vi "Test.vi"() -> ()   [LabVIEW 2012]
doc: "This example shows how to read values from a digital channel.\n\nIt will display the digital value as Low (LED off) or High (LED on).\n\nThis example works with the NI 9403 module connected to a Digital Sidecar. The Digital Sidecar should have 12V applied to the WAGO connector. Note that the digital channels are pulled high when floating. This means that if you want to read a limit switch, you would need to connect one end of the switch to SIG and the other end to (-). The the LED would be On when the switch is open and Off when the switch is closed."
uses:
  <vilib>/Rock Robotics/SystemInterfaces/Typedef/FPGA_TypedefDigitalModule.ctl
  <vilib>/Rock Robotics/WPI/Relay/WPI_RelayDirection.ctl
  <vilib>/Rock Robotics/SystemInterfaces/Utilities/FPGA_UtilitiesLED Source.ctl
  <vilib>/Rock Robotics/SystemInterfaces/Utilities/FPGA_UtilitiesLED State.ctl
  <vilib>/Rock Robotics/WPI/MotorControl/WPI_MotorControlOpen Victor.vi
panel:
  out "PWM":bool[](array[boolean])
  in  "PWM Out":dbl(knob) scale=-1.0..1.0
  in  "Foward":bool
  out "Relay":T1
  out "DIO":bool[](array[boolean])
  out "Beacon\nLight":bool
  in  "DIO Module":T2
  in  "stop":bool
  # "I2C"
  # "Set these inputs before running."
  # "Green/Foward is Signal 5 V"
  # "Red / Reverse is Power 5V"
  # "DIO 1"
  # "DIO 2"
  # "Digital Side Car"
  # "DIO 3"
  # "DIO 4"
  # "DIO 5"
  # "DIO 6"
  # "DIO 7"
  # "DIO 8"
  # "DIO 9"
  # "DIO 10"
  # "DIO 11"
  # "DIO  12"
  # "DIO 13"
  # "DIO 14"
  # "DIO 1"
  # "DIO 2"
  # "DIO 3"
  # "DIO 4"
  # "DIO 5"
  # "DIO 6"
  # "DIO 7"
  # "DIO 8"
  # "DIO 9"
  # "DIO 10"
  # "Reverse"
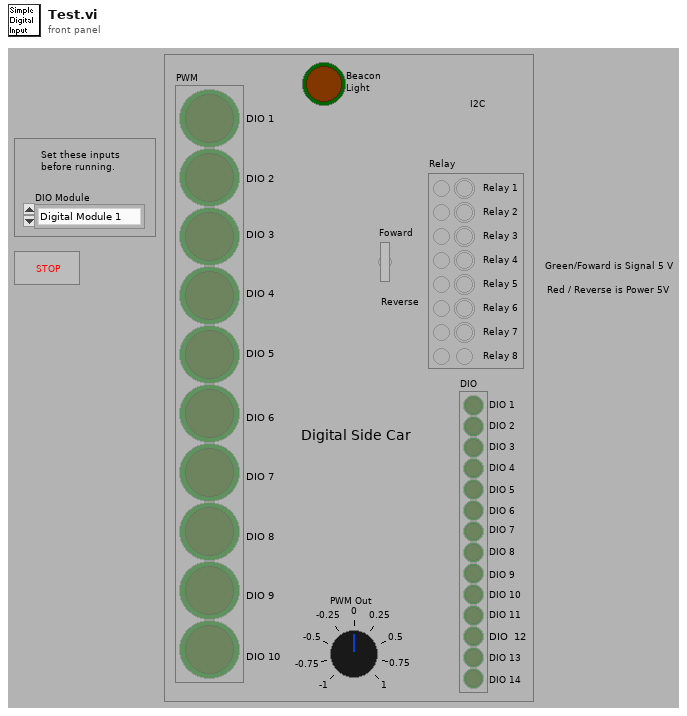
[diagram p1: front panel]
types:
  T1 = cluster{"Relay 1":bool, "Boolean":bool, "Boolean 2":bool, "Relay 2":bool, "Boolean 3":bool, "Relay 3":bool, "Boolean 4":bool, "Relay 4":bool, "Boolean 5":bool, "Relay 5":bool, "Boolean 6":bool, "Relay 6":bool, "Boolean 7":bool, "Relay 7":bool, "Boolean 8":bool, "Relay 8":bool}
  T2 = typedef "FPGA_TypedefDigitalModule.ctl" = enum16{"Digital Module 1", "Digital Module 2"}
  T3 = typedef "WPI_MotorControlDeviceRef.ctl" = cluster{"DeviceStatus":errorcluster, "Type":enum16{"PWM", "CAN"}, "PWM":cluster{"Digital Module":T2, "PWM Channel":T4, "DeadBand":T5}, "CAN":cluster{"Device Number":u8, "Control Mode":T6, "Semaphore":T7, "Max Vout":dbl}, "Invert":bool, "TransformRef":T8, "InvTransformRef":T8}
  T4 = typedef "FPGA_DIOPWMChannel.ctl" = enum8{"PWM 1", "PWM 2", "PWM 3", "PWM 4", "PWM 5", "PWM 6", "PWM 7", "PWM 8", "PWM 9", "PWM 10", "Invalid"}
  T5 = typedef "WPI_PWMDeadband.ctl" = cluster{"Name":string, "maxPositivePwm":i32, "minPositivePwm":i32, "centerPwm":i32, "maxNegativePwm":i32, "minNegativePwm":i32, "angularRange":u16}
  T6 = typedef "WPI_CANJaguar_ControlMode.ctl" = enum8{"Percent VBus", "Current", "Speed", "Position", "Voltage"}
  T7 = typedef "Semaphore RefNum" = refnum<k1>
  T8 = typedef "WPI_PWMTransform_ConPane.ctl" = refnum<vi>
  T9 = typedef "WPI_DigitalInputDevRef.ctl" = cluster{"DevStatus":errorcluster, "DIO Channel":T10, "Digital Module":T2}
  T10 = typedef "FPGA_DIOChannel.ctl" = enum8{"DIO 1", "DIO 2", "DIO 3", "DIO 4", "DIO 5", "DIO 6", "DIO 7", "DIO 8", "DIO 9", "DIO 10", "DIO 11", "DIO 12", "DIO 13", "DIO 14", "Invalid"}
  T11 = typedef "WPI_RelayDirection.ctl" = enum16{"Both directions", "Forward only", "Reverse only"}
  T12 = typedef "WPI_RelayDevRef.ctl" = cluster{"DevStatus":errorcluster, "Relay Channel":T13, "Digital Module":T2, "Relay Direction":T11}
  T13 = typedef "FPGA_DIORelayChannel.ctl" = enum8{"Relay 1", "Relay 2", "Relay 3", "Relay 4", "Relay 5", "Relay 6", "Relay 7", "Relay 8", "Invalid"}
  T14 = typedef "FPGA_UtilitiesLED State.ctl" = enum16{"Off", "On", "Toggle"}
  T15 = typedef "FPGA_UtilitiesLED Source.ctl" = enum16{"User LED", "FPGA LED"}
  T16 = cluster{bool, bool, bool, bool, bool, bool, bool, bool, bool, bool, bool, bool, bool, bool, bool, bool}
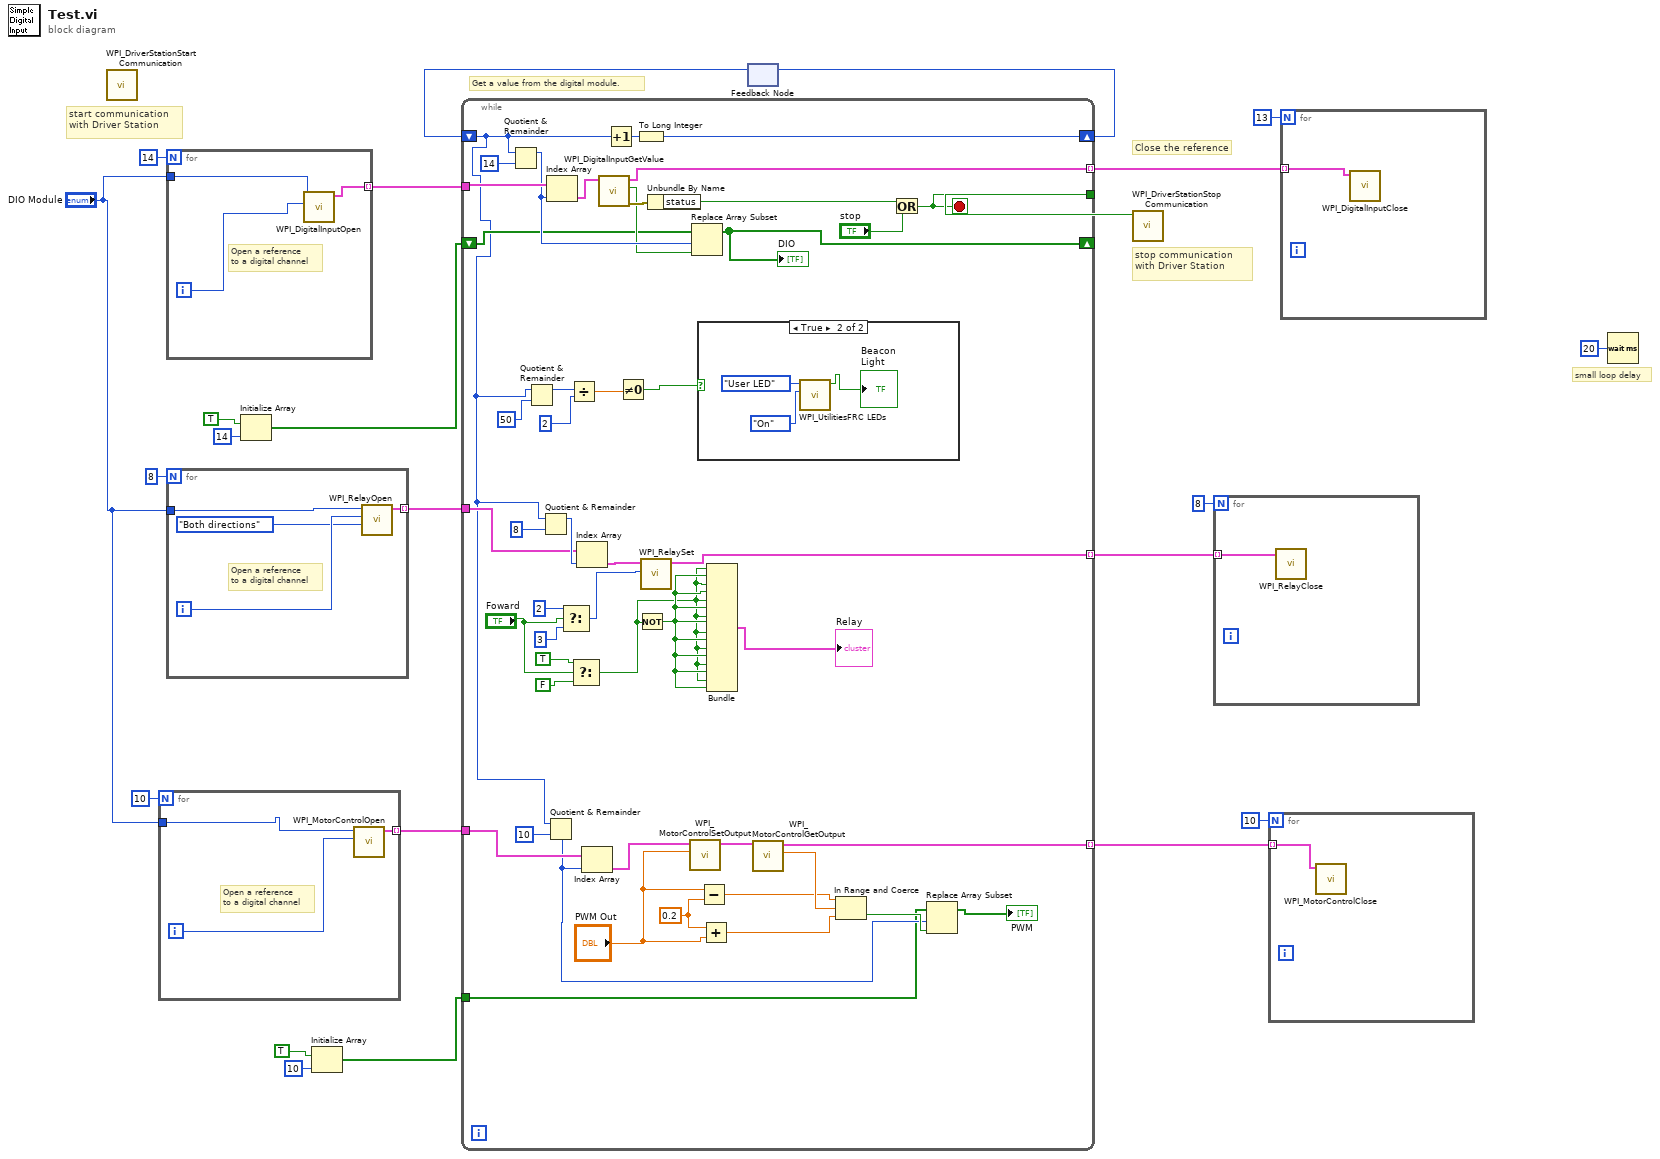
[diagram p0: block diagram]
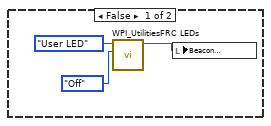
[diagram p2: hidden frame]
diagram:
  # "Get a value from the digital module."
  # "small loop delay"
  # "stop communication with Driver Station"
  # "start communication with Driver Station"
  # "Close the reference"
  n1 = call <vilib>:"WPI_DriverStationStart Communication.vi"() -> ()  [unwired: 1 in, 11 out]
  n2 = for {
    N: 10 -> [_]
    tunnel: [w25] -> w7 mode=indexing
    tunnel: "DIO Module" -> [w24]
    i -> [w26]
    # "Open a reference\nto a digital channel"
    n3 = call-poly <vilib>:"WPI_MotorControlOpen.vi"("PWM Channel"=w26, "Digital Module (Module 1)"=w24) -> ("MotorControlDeviceRef"=w25:T3)  [unwired: 8 in, 1 out]
  }
  n4 = for {
    N: 14 -> [_]
    tunnel: [w29] -> w21 mode=indexing
    tunnel: "DIO Module" -> [w27]
    i -> [w28]
    # "Open a reference\nto a digital channel"
    n5 = call <vilib>:"WPI_DigitalInputOpen.vi"("DIO Channel"=w28, "Digital Module (Module 1)"=w27) -> ("DigitalInputDevRef"=w29:T9)  [unwired: 1 in, 8 out]
  }
  n6 = for {
    N: 8 -> [_]
    tunnel: [w31] -> w11 mode=indexing
    tunnel: "DIO Module" -> [w30]
    i -> [w33]
    # "Open a reference\nto a digital channel"
    n7 = call <vilib>:"WPI_RelayOpen.vi"("Relay Direction"=WPI_RelayDirection."Both directions", "Relay Channel"=w33, "Digital Module (Module 1)"=w30) -> ("RelayDevRef"=w31:T12)  [unwired: 7 in, 1 out]
  }
  n8 = Initialize Array(TRUE, 14 ("dimension size")) -> (w15:bool[])
  n9 = Initialize Array(TRUE, 10 ("dimension size")) -> (w4:bool[])
  n10 = feedback #1() -> (w18:i32)  [unwired: 1 in]
  n11 = while {
    tunnel: [w80] -> w23
    tunnel: w21 -> [w73]
    shift-right: [w75] -> w19
    shift-left: w18 -> [w50]
    shift-right: [w69] -> _
    shift-left: w15 -> [w70]
    tunnel: [w68] -> w13 mode=indexing
    tunnel: w11 -> [w65]
    tunnel: [w57] -> w9 mode=indexing
    tunnel: w7 -> [w49]
    tunnel: w4 -> [w38]
    tunnel: [w34] -> w1 mode=indexing
    stop <- w80 stop-if-true
    w42 = 0.2
    n12 = Quotient & Remainder(x=w50, y=14) -> (x-y*floor(x/y)=w72:i32)  [unwired: 1 out]
    n13 = Quotient & Remainder(x=w50, y=50) -> (x-y*floor(x/y)=w55:i32)  [unwired: 1 out]
    n14 = Quotient & Remainder(x=w50, y=8) -> (x-y*floor(x/y)=w66:i32)  [unwired: 1 out]
    n15 = Quotient & Remainder(x=w50, y=10) -> (x-y*floor(x/y)=w39:i32)  [unwired: 1 out]
    n16 = Index Array(array=w73, index=w72) -> (element=w74:T9)
    n17 = Select(t=2, s="Foward", f=3 ("t")) -> (s? t:f=w61:i32)
    n18 = Divide(x=w55, y=2) -> (x/y=w52:dbl)
    n19 = Select(t=TRUE, s="Foward", f=FALSE) -> (s? t:f=w35:bool)
    n20 = Index Array(array=w65, index=w66) -> (element=w64:T12)
    n21 = Index Array(array=w49, index=w39) -> (element=w48:T3)
    n22 = call <vilib>:"WPI_DigitalInputGetValue.vi"("DigitalInputDevRef"=w74) -> ("error out"=w79:errorcluster, "Value"=w71:bool, "DigitalInputDevRef"=w68:T9)  [unwired: 1 in, 7 out]
    n23 = Increment(x=w50) -> (x+1=w77:i32)
    n24 = Not Equal To 0?(x=w52) -> (x != 0?=w53:bool)
    n25 = To Long Integer(number=w77) -> (32bit integer=w75:i32)
    n26 = Not(x=w35) -> (.not. x?=w36:bool)
    n27 = call <vilib>:"WPI_RelaySet.vi"("RelayValue"=w61, "RelayDevRef"=w64) -> ("RelayDevRef"=w57:T12)  [unwired: 8 in, 1 out]
    n28 = Unbundle By Name(w79) -> ("status"=w81:bool)
    n29 = call <vilib>:"WPI_MotorControlSetOutput.vi"("Output"="PWM Out", "MotorControlDevRef"=w48) -> ("MotorControlDevRef"=w47:T3)  [unwired: 7 in, 2 out]
    n30 = Replace Array Subset(array=w70, new element=w71, index=w72) -> (w69:bool[])
    "DIO" <- w69
    n31 = case shown="True" w53 {
      frame False {
        n32 = call <vilib>:"WPI_UtilitiesFRC LEDs.vi"("State"=FPGA_UtilitiesLED_State."Off", "LED Type"=FPGA_UtilitiesLED_Source."User LED") -> ("LED State"=w82:bool)  [unwired: 8 in, 1 out]
        n33 = local write "Beacon\nLight"(w82) -> ()
      }
      frame True {
        n34 = call <vilib>:"WPI_UtilitiesFRC LEDs.vi"("State"=FPGA_UtilitiesLED_State."On", "LED Type"=FPGA_UtilitiesLED_Source."User LED") -> ("LED State"=→"Beacon\nLight":bool)  [unwired: 8 in, 1 out]
      }
    }
    n35 = Subtract(x="PWM Out", y=w42) -> (x-y=w43:dbl)
    n36 = Add(x=w42, y="PWM Out") -> (x+y=w44:dbl)
    n37 = Bundle(w35, w36, w35, w36, w35, w36, w35, w36, w35, w36, w35, w36, w35, w36, w35, w36) -> (→"Relay":T16)  [unwired: 1 in]
    n38 = call <vilib>:"WPI_MotorControlGetOutput.vi"("MotorControlDevRef"=w47) -> ("Output"=w46:dbl, "MotorControlDevRef"=w34:T3)  [unwired: 8 in, 1 out]
    n39 = In Range and Coerce(upper limit=w43, x=w46, lower limit=w44) -> (In Range?=w40:bool)  [unwired: 1 out]
    n40 = Or(x=w81, y="stop") -> (x .or. y?=w80:bool)
    n41 = Replace Array Subset(array=w38, new element=w40, index=w39) -> (→"PWM":bool[])
  }
  n42 = feedback-in #1(w19) -> ()
  n43 = call <vilib>:"WPI_DriverStationStop Communication.vi"("StopCommunication"=w23) -> ()  [unwired: 1 in, 10 out]
  n44 = for {
    N: 8 -> [_]
    tunnel: w9 -> [w88] mode=indexing
    n45 = call <vilib>:"WPI_RelayClose.vi"("RelayDevRef"=w88) -> ()  [unwired: 10 in, 1 out]
  }
  n46 = for {
    N: 10 -> [_]
    tunnel: w1 -> [w89] mode=indexing
    n47 = call <vilib>:"WPI_MotorControlClose.vi"("MotorControlDevRef"=w89) -> ()  [unwired: 10 in, 1 out]
  }
  n48 = for {
    N: 13 -> [_]
    tunnel: w13 -> [w90] mode=indexing
    n49 = call <vilib>:"WPI_DigitalInputClose.vi"("DigitalInputDevRef"=w90) -> ()  [unwired: 1 in, 10 out]
  }
  n50 = Wait (ms)(milliseconds to wait=u32 20) -> ()  [unwired: 1 out]
